vi "Hide Splash.vi"(8 "error in (no error)":errorcluster, 11 "Volatus Core in":refnum<class "Volatus Core.lvclass">) -> (0 "error out":errorcluster, 3 "Volatus Core out":refnum<class "Volatus Core.lvclass">)   [LabVIEW 2020, in "Volatus.lvlib" / "Volatus Core.lvclass"]
uses:
  Volatus Core.lvclass
  Volatus Core.lvclass/Volatus Core.ctl
  Splash Screen/Splash Screen.lvclass
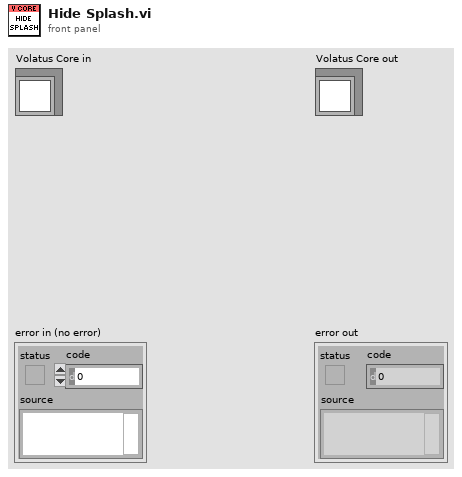
[diagram p1: front panel]
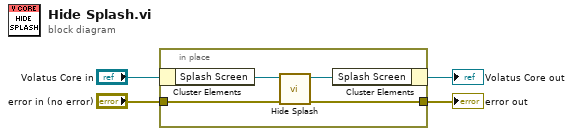
[diagram p0: block diagram]
diagram:
  n1 = in-place {
    in-place-border: "error in (no error)" -> [w7]
    in-place-border: [w5] -> w1
    n2 = in-place-cluster #1("Volatus Core in") -> ("Splash Screen"=w8:refnum<class "Splash Screen.lvclass">)
    n3 = call-dynamic "Hide Splash.vi"("error in (no error)"=w7, "Splash Screen in"=w8) -> ("error out"=w5:errorcluster, "Splash Screen out"=w6:refnum<class "Splash Screen.lvclass">)  [unwired: 8 in]
    n4 = in-place-cluster #1("Splash Screen"=w6) -> (→"Volatus Core out":refnum<class "Volatus Core.lvclass">)
  }
  "error out" <- w1
